vi "dosimat876_write_command.vi"(3 "error in":errorcluster, 4 "write buffer":string, 5 "Dosimat Port In":refnum<visa-resource-name>="COM1") -> (0 "error out":errorcluster, 1 "read buffer":string, 2 "Dosimat Port Out":refnum<visa-resource-name>="COM1")   [LabVIEW 2010]
uses:
  <vilib>/Instr/_visa.llb/VISA Configure Serial Port (Instr).vi
panel:
  # "mooseNote: tell it which of the commands \nto write and it will send it to the 876"
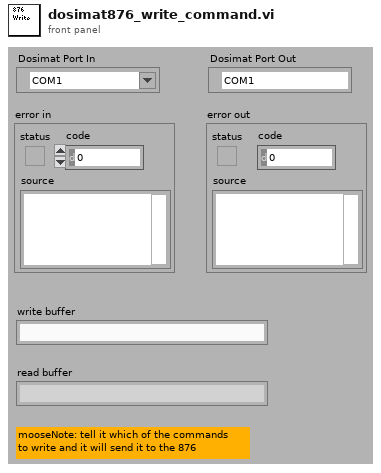
[diagram p1: front panel]
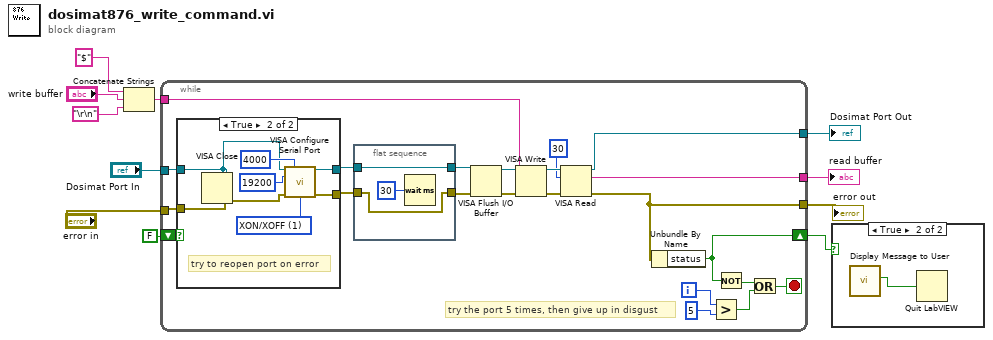
[diagram p0: block diagram]
diagram:
  n1 = Concatenate Strings("$" ("string"), "write buffer", "\r\n") -> (w9:string)
  n2 = while {
    tunnel: w9 -> [w31]
    tunnel: "error in" -> [w24]
    tunnel: "Dosimat Port In" -> [w25]
    shift-right: [w12] -> w1
    shift-left: FALSE -> [w23]
    tunnel: [w20] -> w4
    tunnel: [w15] -> w3
    tunnel: [w19] -> w2
    i -> [w13]
    stop <- w16 stop-if-true
    # "try the port 5 times, then give up in disgust"
    n3 = case shown="True" w23 {
      tunnel: [w35 w37] -> w22
      tunnel: w25 -> [w35 w39]
      tunnel: [w34 w36] -> w21
      tunnel: w24 -> [w34 w43]
      frame False {
      }
      frame True {
        w41 = u16 1 items=["None", "XON/XOFF", "RTS/CTS", "XON/XOFF & RTS/CTS", "DTR/DSR", "XON/XOFF & DTR/DSR"] ("flow control (0:none)")
        # "try to reopen port on error"
        n4 = VISA Close(VISA resource name=w39, error in (no error)=w43) -> (error out=w38:errorcluster)
        n5 = call-poly "VISA Configure Serial Port"("VISA resource name"=w39, "timeout (10sec)"=u32 4000, "baud rate (9600)"=u32 19200, "error in (no error)"=w38, "flow control (0:none)"=w41) -> ("VISA resource name out"=w37:refnum<visa-resource-name>, "error out"=w36:errorcluster)  [unwired: 9 in]
      }
    }
    n6 = flat-sequence {
      tunnel: [w44] -> w27
      tunnel: w21 -> [w45]
      tunnel: [w45] -> w26
      tunnel: w22 -> [w44]
      frame #0 {
        n7 = Wait (ms)(milliseconds to wait=u32 30) -> ()  [unwired: 1 out]
      }
    }
    n8 = VISA Flush I/O Buffer(VISA resource name=w27, error in (no error)=w26) -> (VISA resource name out=w29:refnum<visa-resource-name>, error out=w28:errorcluster)  [unwired: 1 in]
    n9 = VISA Write(VISA resource name=w29, write buffer=w31, error in (no error)=w28) -> (VISA resource name out=w33:refnum<visa-resource-name>, error out=w32:errorcluster)  [unwired: 1 out]
    n10 = VISA Read(VISA resource name=w33, byte count=u32 30, error in (no error)=w32) -> (VISA resource name out=w20:refnum<visa-resource-name>, read buffer=w19:string, error out=w15:errorcluster)  [unwired: 1 out]
    n11 = Unbundle By Name(w15) -> ("status"=w12:bool)
    n12 = Greater?(x=w13, y=5) -> (0:w18:bool)
    n13 = Not(x=w12) -> (.not. x?=w17:bool)
    n14 = Or(x=w17, y=w18) -> (x .or. y?=w16:bool)
  }
  "Dosimat Port Out" <- w4
  "error out" <- w3
  "read buffer" <- w2
  n15 = case shown="True" w1 {
    frame False {
    }
    frame True {
      n16 = call "Display Message to User"() -> ("OK"=w47:bool)  [unwired: 10 in, 1 out]
      n17 = Quit LabVIEW(quit? (T)=w47) -> ()
    }
  }
